vi "Do.vi"(8 "error in (no error)":errorcluster, 10 "Actor in":refnum<class "Actor.lvclass">, 11 "Show View Msg":refnum<class "Open Front Panel Msg.lvclass">) -> (0 "error out":errorcluster, 2 "Actor out":refnum<class "Actor.lvclass">)   [LabVIEW 2020, in "MVA Framework.lvlib" / "IViewable.lvlib" / "Open Front Panel Msg.lvclass"]
doc: "This VI delivers the message to the actor by calling the appropriate method(s) on the actor.\n\n<License>\nCopyright © 2017 Composed Systems, LLC | All rights reserved\nwww.composed.io\n\nAuthor: Ethan Stern <ethan.stern@composed.io>\n\nThis software is provided \"AS IS\" WITHOUT WARRANTIES, either express or implied, AND IS FOR EDUCATIONAL PURPOSES ONLY.\n</License>"
uses:
  Open Front Panel Msg.lvclass
  <vilib>/ActorFramework/Actor/Actor.lvclass
  IViewable/IViewable.lvclass
  C:/Program Files/National Instruments/LabVIEW 2020/vi.lib/ActorFramework/Actor/Actor.lvclass
  Open Front Panel Msg.lvclass/Open Front Panel Msg.ctl
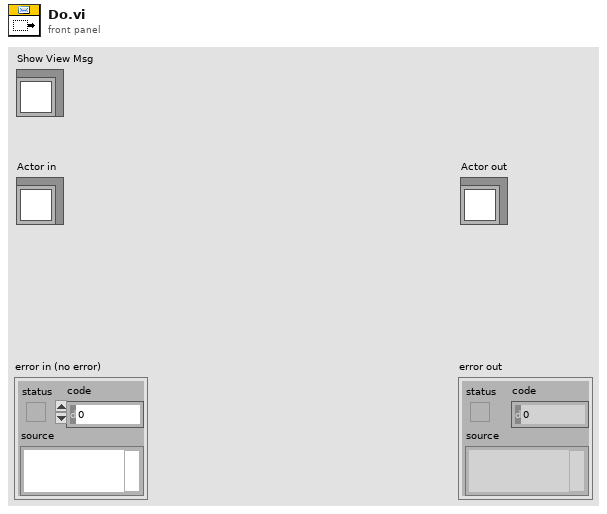
[diagram p1: front panel]
types:
  T1 = typedef "MVA Framework.lvlib/IViewable.lvlib/IViewable.lvclass/View Position Enum.ctl" = enum16{"Centered", "Maximized", "Minimized", "Custom", "Unchanged"}
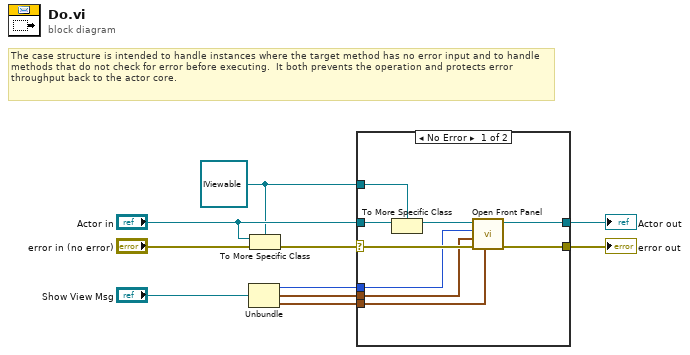
[diagram p0: block diagram]
diagram:
  w4 = refnum<class "IViewable.lvclass"> refnum ("Actor in")
  # "The case structure is intended to handle instances where the target method has no error input and to handle methods that do not check for error before executing.  It both prevents the operation and protects error throughput back to the actor core."
  n1 = Unbundle("Show View Msg") -> (w3:T1, w2:cluster{"Top":i16, "Left":i16}, w1:cluster{"Height":i16, "Width":i16})
  n2 = To More Specific Class(target class=w4, reference="Actor in", error in="error in (no error)") -> (error out=w8:errorcluster)  [unwired: 1 out]
  n3 = case shown="No Error" w8 {
    selector: w8 -> [w17 w21]
    tunnel: [w19 w21] -> w7
    tunnel: [w18 w20] -> w6
    tunnel: "Actor in" -> [w16 w20]
    tunnel: w4 -> [w15 _]
    tunnel: w3 -> [w13 _]
    tunnel: w2 -> [w12 _]
    tunnel: w1 -> [w11 _]
    frame No Error {
      n4 = To More Specific Class(target class=w15, reference=w16) -> (specific class reference=w14:refnum<class "IViewable.lvclass">)  [unwired: 1 in, 1 out]
      n5 = call-dynamic "Open Front Panel.vi"("Custom Window Size"=w11, "error in (no error)"=w17, "Custom Window Position"=w12, "Position"=w13, "IViewable in"=w14) -> ("error out"=w19:errorcluster, "IViewable out"=w18:refnum<class "IViewable.lvclass">)  [unwired: 5 in]
    }
    frame Error {
      # "If type check fails, pass the\noriginal object out again."
    }
  }
  "error out" <- w7
  "Actor out" <- w6
